vi "Write Fluidics Active.vi"(8 "error in (no error)":errorcluster, 10 "Fluidics Active":bool, 11 "Main Window in":refnum<class "Main Window.lvclass">) -> (0 "error out":errorcluster, 3 "Main Window out":refnum<class "Main Window.lvclass">)   [LabVIEW 2015, in "Main Window.lvlib" / "Main Window.lvclass"]
uses:
  Main Window.lvclass
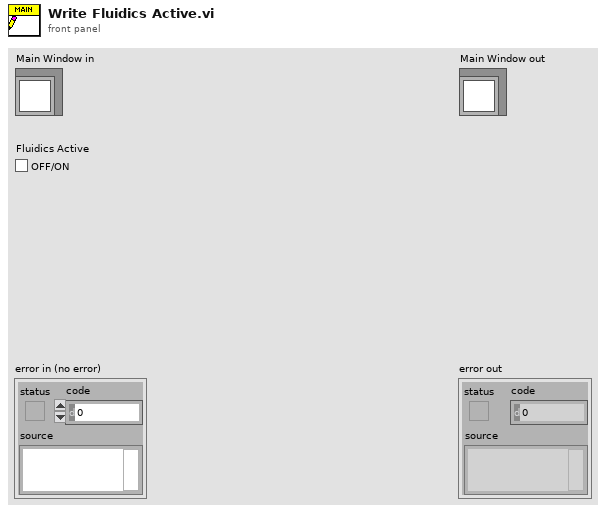
[diagram p1: front panel]
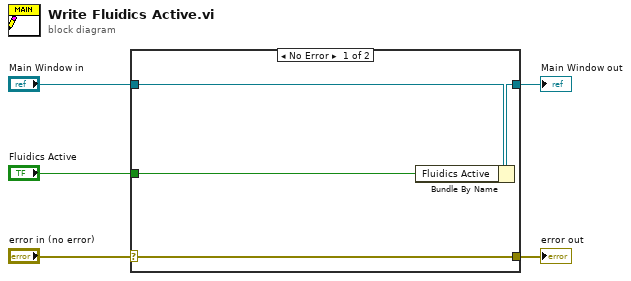
[diagram p0: block diagram]
diagram:
  n1 = case shown="No Error" "error in (no error)" {
    selector: "error in (no error)" -> [w9 w10]
    tunnel: [w9 w10] -> w4
    tunnel: [w7 w11] -> w2
    tunnel: "Main Window in" -> [w8 w11]
    tunnel: "Fluidics Active" -> [w6 _]
    frame No Error {
      n2 = Bundle By Name(cluster=w8, "Fluidics Active"=w6) -> (w7:refnum<class "Main Window.lvclass">)
    }
    frame Error {
    }
  }
  "error out" <- w4
  "Main Window out" <- w2
